vi "ast_reql_query_set.vi"(8 "error in (no error)":errorcluster, 10 "query":string, 11 "reql_id in":u32 format="%08x") -> (0 "error out":errorcluster, 3 "reql_id out":u32 format="%08x")   [LabVIEW 2017]
uses:
  ast_reql_cache_action.ctl
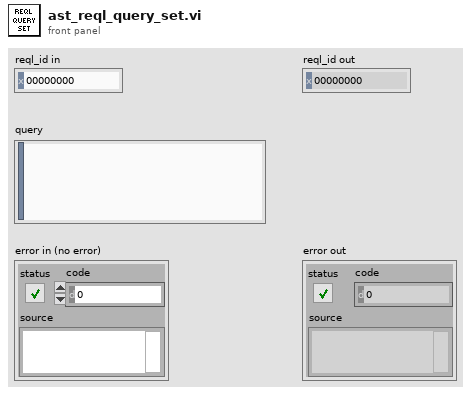
[diagram p1: front panel]
types:
  T1 = typedef "ast_reql_cache_action.ctl" = enum8{"null", "new", "get_query", "get_response", "set_query", "set_response", "delete"}
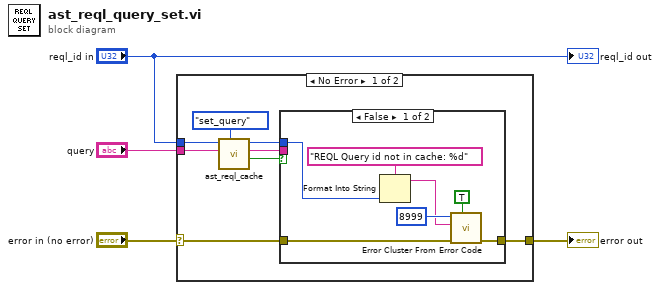
[diagram p0: block diagram]
diagram:
  n1 = case shown="No Error" "error in (no error)" {
    selector: "error in (no error)" -> [w7 w21]
    tunnel: "reql_id in" -> [w6 _]
    tunnel: [w8 w21] -> w4
    tunnel: "query" -> [w5 _]
    frame No Error {
      n2 = call "ast_reql_cache.vi"("action"=ast_reql_cache_action."set_query", "query in"=w5, "reql_id in"=w6) -> ("exists?"=w10:bool, "query out"=w9:string, "reql_id out"=w11:u32)  [unwired: 6 in]
      n3 = case shown="False" w10 {
        tunnel: w11 -> [w13 _]
        tunnel: w9 -> [_ _]
        tunnel: [w18 w20] -> w8
        tunnel: w7 -> [w19 w20]
        frame False {
          n4 = Format Into String(format string="REQL Query id not in cache: %d" ("error message (\"\")"), w13) -> (resulting string=w14:string)  [unwired: 2 in, 1 out]
          n5 = call <vilib>:"Error Cluster From Error Code.vi"("show call chain? (False)"=TRUE, "error in (no error)"=w19, "error message (\"\")"=w14, "error code (0)"=8999) -> ("error out"=w18:errorcluster)  [unwired: 5 in]
        }
        frame True {
        }
      }
    }
    frame Error {
    }
  }
  "error out" <- w4
  "reql_id out" <- "reql_id in"
